vi "断电保存全局.vi"() -> ()   [LabVIEW 2022 SP3, in "超标留样集成.lvlib"]
panel:
  out "初始化":bool
  in  "PH下限浓度":dbl
  in  "汞超标浓度":dbl
  in  "锰超标浓度":dbl
  in  "镍超标浓度":dbl
  in  "锌超标浓度":dbl
  in  "铜超标浓度":dbl
  in  "镉超标浓度":dbl
  in  "铅超标浓度":dbl
  in  "COD超标浓度":dbl
  in  "ORP超标浓度":dbl
  in  "藻密度超标浓度":dbl
  in  "蓝绿藻超标浓度":dbl
  in  "叶绿素a超标浓度":dbl
  in  "浊度超标浓度":dbl
  in  "SPCOND超标浓度":dbl
  in  "DO超标浓度":dbl
  in  "PH超标浓度":dbl
  in  "CODCr超标浓度":dbl
  in  "CODMn超标浓度":dbl
  in  "总氮超标浓度":dbl
  in  "总磷超标浓度":dbl
  in  "氨氮超标浓度":dbl
  in  "超标留样型号":T1(ring)
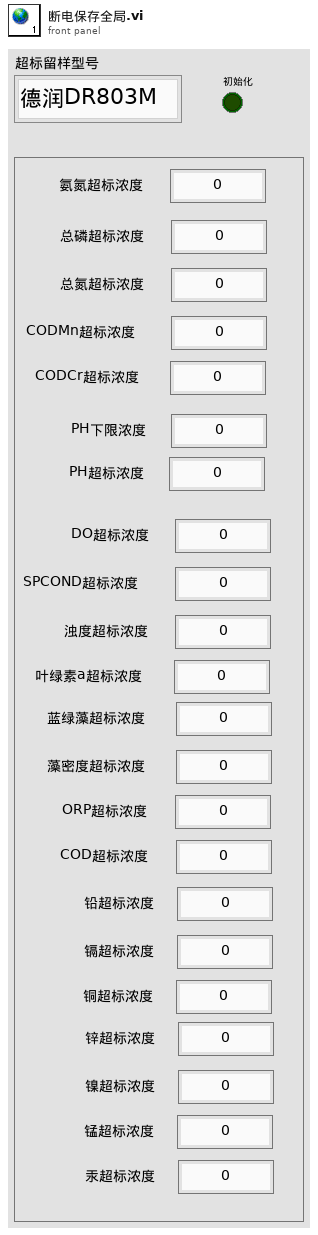
[diagram p1: front panel]
types:
  T1 = enum16{"德润DR803M", "德润DR803L", "德润DR803F", "科盛超标留样", "德润DR803M4", "ESTD1200"}
diagram:
